vi "Discovery Client FGV.vi"(8 "error in":errorcluster, 10 "unique id in":u64, 11 "action":T2) -> (0 "error out":errorcluster, 1 "cluster id":string, 2 "unique id out":u64, 3 "grpc client id":T1)   [LabVIEW 2020, in "NI Discovery V1 Client.lvlib"]
uses:
  NI Discovery V1 Client.lvlib
  TypeDefs/gRPC Client Cache FGV Action.ctl
  <vilib>/gRPC/LabVIEW gRPC Library/Shared/grpcId.ctl
  TypeDefs/gRPC Client Cache VI References.ctl
  Create Client.vi
  Recreate Client.vi
  <vilib>/gRPC/LabVIEW gRPC Library/grpc-lvsupport-release.lvlib
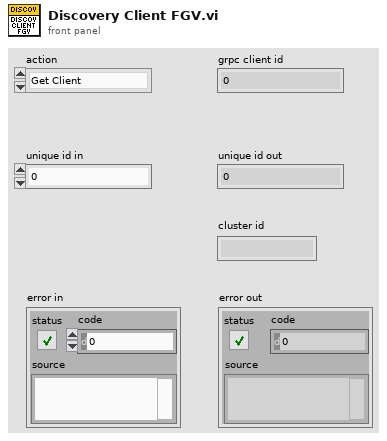
[diagram p1: front panel]
types:
  T1 = typedef "grpc-lvsupport-release.lvlib/grpcId.ctl" = u64
  T2 = typedef "NI Discovery V1 Client.lvlib/gRPC Client Cache FGV Action.ctl" = enum16{"Get Client", "Recreate Client", "Destroy Client", "Update ClusterId"}
  T3 = typedef "NI Discovery V1 Client.lvlib/gRPC Client Cache VI References.ctl" = cluster{"create vi reference":refnum<vi>, "recreate vi reference":refnum<vi>}
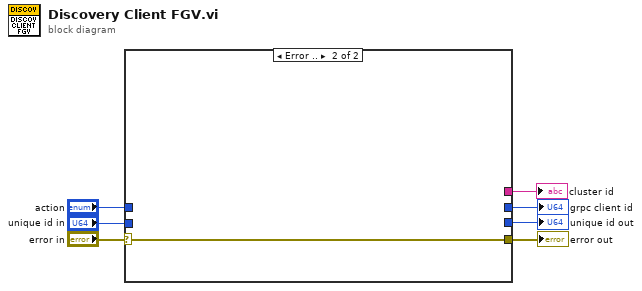
[diagram p0: block diagram]
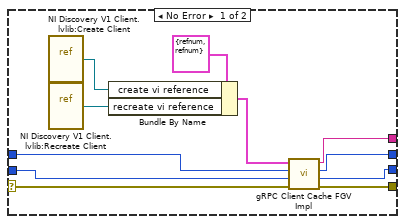
[diagram p2: hidden frame]
diagram:
  n1 = case shown="Error .." "error in" {
    selector: "error in" -> [w18 w19]
    tunnel: [w15 w19] -> w7
    tunnel: "action" -> [w17 _]
    tunnel: [w14 _] -> w6
    tunnel: "unique id in" -> [w16 _]
    tunnel: [w13 _] -> w2
    tunnel: [w8 _] -> w1
    frame No Error {
      n2 = vi-ref "NI Discovery V1 Client.lvlib:Create Client.vi"() -> (w11:refnum<vi>)
      n3 = vi-ref "NI Discovery V1 Client.lvlib:Recreate Client.vi"() -> (w9:refnum<vi>)
      n4 = Bundle By Name(cluster=T3 {"create vi reference"=refnum, "recreate vi reference"=refnum} ("vi references in"), "create vi reference"=w11, "recreate vi reference"=w9) -> (w10:T3)
      n5 = call "gRPC Client Cache FGV Impl.vi"("error in"=w18, "unique id in"=w16, "action"=w17, "vi references in"=w10) -> ("error out"=w15:errorcluster, "unique id out"=w13:u64, "grpc client id"=w14:T1, "cluster id"=w8:string)  [unwired: 4 in]
    }
    frame Error {
    }
  }
  "error out" <- w7
  "grpc client id" <- w6
  "unique id out" <- w2
  "cluster id" <- w1
